vi "Write Value.vi"(8 "error in (no error)":errorcluster, 10 "Value":dbl, 11 "Double D Element in":refnum<class "Double D Element.lvclass">) -> (0 "error out":errorcluster, 3 "Double D Element out":refnum<class "Double D Element.lvclass">)   [LabVIEW 2018, in "D Datagrid Library.lvlib" / "Double D Element.lvclass"]
uses:
  Double D Element.lvclass
  Double D Element.lvclass/Double D Element.ctl
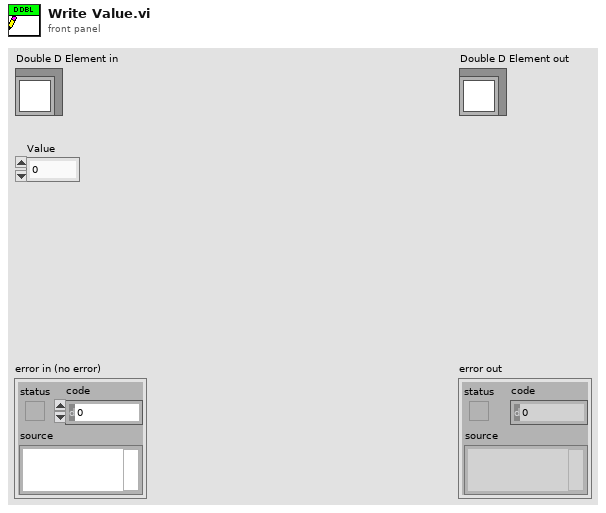
[diagram p1: front panel]
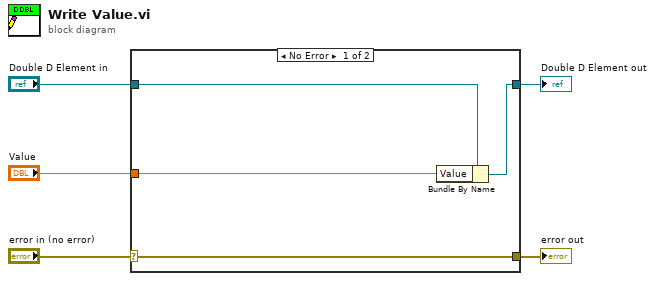
[diagram p0: block diagram]
diagram:
  n1 = case shown="No Error" "error in (no error)" {
    selector: "error in (no error)" -> [w9 w10]
    tunnel: [w9 w10] -> w4
    tunnel: [w7 w11] -> w2
    tunnel: "Double D Element in" -> [w8 w11]
    tunnel: "Value" -> [w6 _]
    frame No Error {
      n2 = Bundle By Name(cluster=w8, "Value"=w6) -> (w7:refnum<class "Double D Element.lvclass">)
    }
    frame Error {
    }
  }
  "error out" <- w4
  "Double D Element out" <- w2
